vi "waveform_Graph.vi"() -> ()   [LabVIEW 2020]
panel:
  out "Waveform Graph":dynamicdata(graph)
  in  "stop":bool
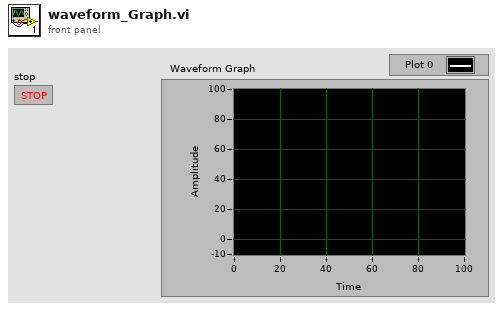
[diagram p1: front panel]
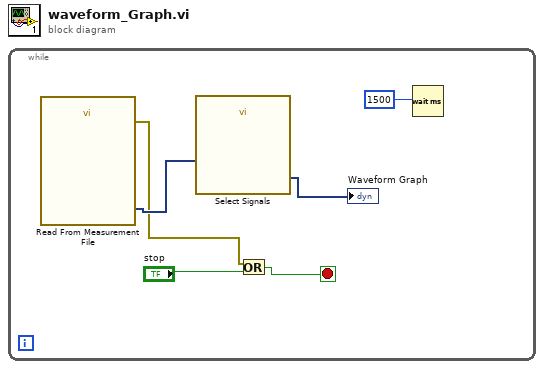
[diagram p0: block diagram]
diagram:
  n1 = while {
    stop <- w5 stop-if-true
    n2 = call "Read From Measurement File"() -> ("error out"=w1:errorcluster, "Signals"=w3:dynamicdata)  [unwired: 6 in, 4 out]
    n3 = call "Select Signals"("Signals"=w3) -> ("Signal Out"=→"Waveform Graph":dynamicdata)  [unwired: 9 in, 1 out]
    n4 = Or(x=w1, y="stop") -> (x .or. y?=w5:bool)
    n5 = Wait (ms)(milliseconds to wait=1500) -> ()  [unwired: 1 out]
  }
